vi "Pre Launch Init.vi"(11 "CoolAppProcess in":refnum<class "CoolAppProcess.lvclass">) -> (0 "error out":errorcluster, 3 "CoolAppProcess out":refnum<class "CoolAppProcess.lvclass">)   [LabVIEW 2020, in "LAF2024Q2.lvlib" / "CoolAppProcess.lvclass"]
doc: "(<B>Filename</B>: Actor Framework.lvlib:Actor.lvclass:Pre Launch Init.vi)\n\nDefines behavior that occurs after the Launch Nested Actor method is invoked but before the actor's Actor Core method begins running.\n\nBy default, this method does nothing. A descendant class may override it to define behavior."
uses:
  CoolAppProcess.lvclass
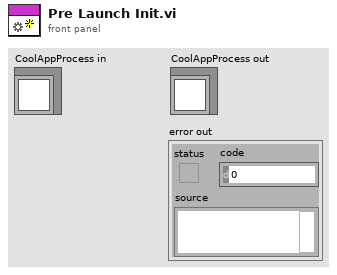
[diagram p1: front panel]
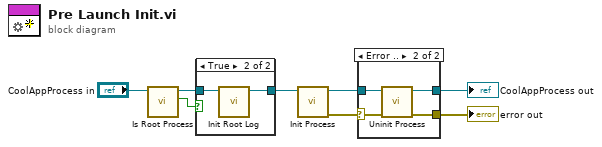
[diagram p0: block diagram]
diagram:
  n1 = call "Is Root Process.vi"("CoolAppProcess in"="CoolAppProcess in") -> ("Root Process"=w3:bool, "CoolAppProcess out"=w2:refnum<class "CoolAppProcess.lvclass">)  [unwired: 8 in, 1 out]
  n2 = case shown="True" w3 {
    tunnel: w2 -> [w9 w11]
    tunnel: [w9 w10] -> w1
    frame False {
    }
    frame True {
      n3 = call "Init Root Log.vi"("CoolAppProcess in"=w11) -> ("CoolAppProcess out"=w10:refnum<class "CoolAppProcess.lvclass">)  [unwired: 9 in, 1 out]
    }
  }
  n4 = call-dynamic "Init Process.vi"("CoolAppProcess in"=w1) -> ("error out"=w7:errorcluster, "CoolAppProcess out"=w5:refnum<class "CoolAppProcess.lvclass">)  [unwired: 9 in]
  n5 = case shown="Error .." w7 {
    selector: w7 -> [w13 w17]
    tunnel: [w13 w16] -> w6
    tunnel: w5 -> [w12 w15]
    tunnel: [w12 w14] -> w4
    frame No Error {
    }
    frame Error {
      n6 = call-dynamic "Uninit Process.vi"("error in (no error)"=w17, "CoolAppProcess in"=w15) -> ("error out"=w16:errorcluster, "CoolAppProcess out"=w14:refnum<class "CoolAppProcess.lvclass">)  [unwired: 8 in]
    }
  }
  "error out" <- w6
  "CoolAppProcess out" <- w4
